vi "AIT 1553 - Parse BC Channels.vi"(6 "Bus Config Info":T10, 7 "FIFO Idx Qs":T12, 8 "error in (no error)":errorcluster, 9 "Bus Page Ref":T1 format="%.0x", 10 "Section GUID":string, 11 "Device Reference in":T1 format="%.0x") -> (0 "error out":errorcluster, 1 "Section BaseRate":u32, 2 "HW Channel - BC Section":T2 {"Message Settings"."Driver Data"."First Word" min=8 max=31; "Message Settings"."Driver Data"."Num Bits" min=1 max=32; "Message Settings"."Driver Data"."Start Bit" min=8 max=31; "Message Settings"."Block Data Refs"."Data Reference" format="%.0x"}, 3 "Device Reference out":T1 format="%.0x", 5 "Bus Controller Page Acyclic Frame Refs out":T1[](array[typedef]) format="%.0x")   [LabVIEW 2013, in "AIT 1553 Custom Device.lvlib"]
uses:
  AIT 1553 Custom Device.lvlib
  <vilib>/NI Veristand/Custom Device API/Custom Device Item Ref.ctl
  RT Controls/FIFO Idx Qs.ctl
  RT Controls/AIT 1553 - Board Config Info.ctl
  RT Controls/AIT 1553 - Hardware Type.ctl
  RT Controls/AIT 1553 - RT HW Channel.ctl
  RT Controls/AIT 1553 - Bus Section.ctl
  RT Controls/AIT 1553 - RT Message Settings.ctl
  <vilib>/NI Veristand/Custom Device API/Block Data Reference.ctl
  <vilib>/NI Veristand/Custom Device API/Data Reference.ctl
  RT Controls/AIT 1553 - Driver Data.ctl
  Controls and Global/Start Bit.ctl
  Controls and Global/Number of Bits.ctl
  <vilib>/NI Veristand/Custom Device Tools/Custom Device Utility Library/RT Debug String Color Spec.ctl
  <vilib>/NI Veristand/Custom Device Tools/Custom Device Utility Library/NI VeriStand - Search for Item by GUID.vi
  Controls and Global/Global.vi
  <vilib>/NI Veristand/Custom Device Tools/Custom Device Utility Library/Custom Device Utility Library.lvlib
  <vilib>/NI Veristand/Custom Device API/Custom Device API.lvlib
  <instrlib>/AIT 1553/AIT 1553.lvlib
  <userlib>/MIL-STD-1553/Owl1553.lvlib
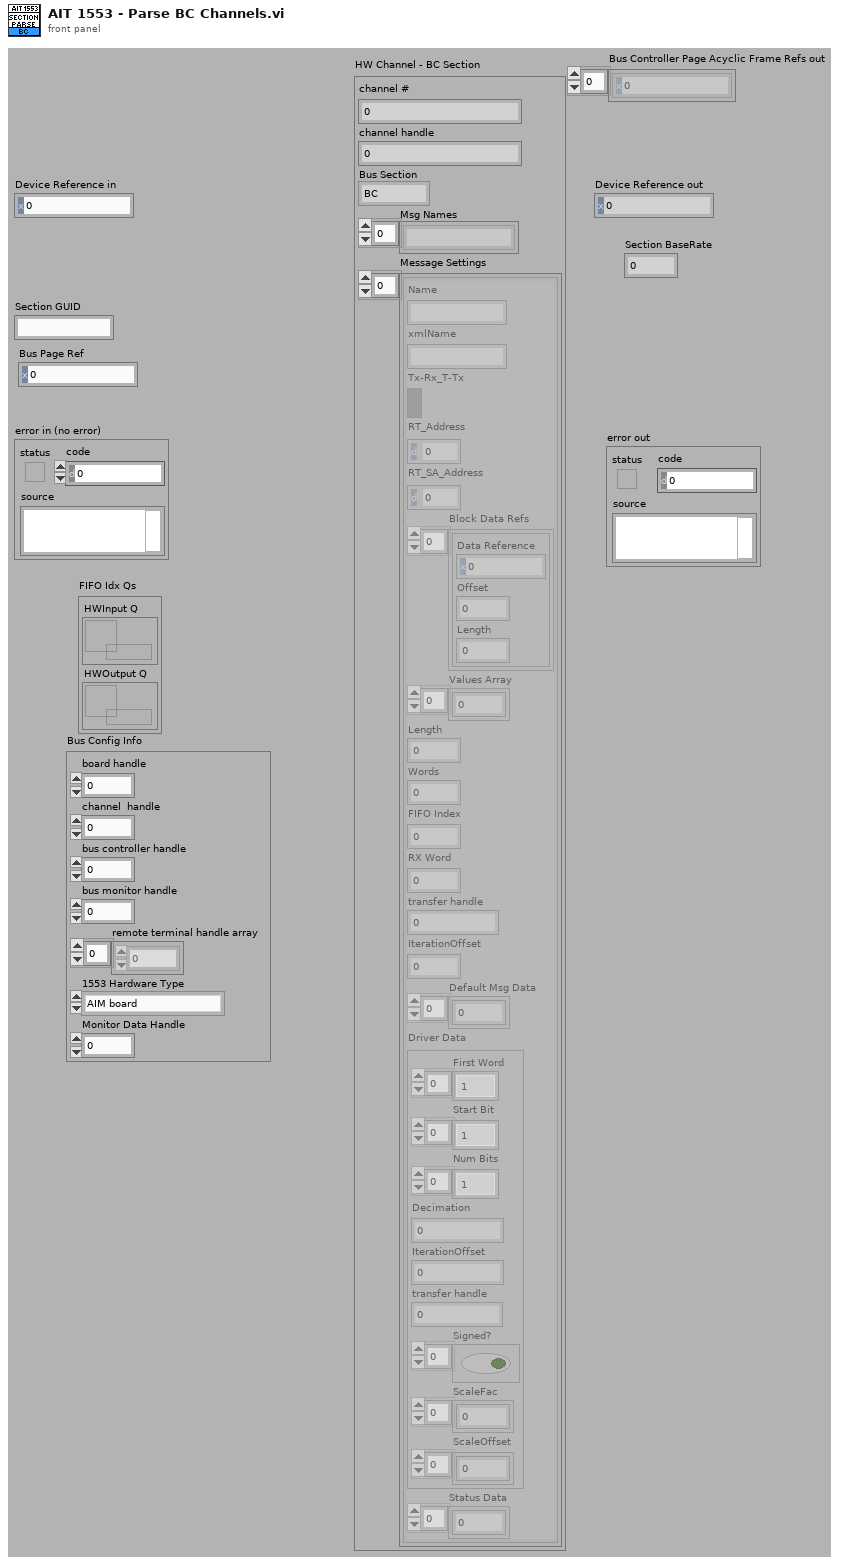
[diagram p1: front panel]
types:
  T1 = typedef "Custom Device API.lvlib/Custom Device Item Ref.ctl" = u64
  T2 = typedef "AIT 1553 Custom Device.lvlib/AIT 1553 - RT HW Channel.ctl" = cluster{"channel #":u16, "channel handle":u32, "Bus Section":T3, "Msg Names":string[], "Message Settings":T4[]}
  T3 = typedef "AIT 1553 Custom Device.lvlib/AIT 1553 - Bus Section.ctl" = enum16{"BC", "BM", "RT"}
  T4 = typedef "AIT 1553 Custom Device.lvlib/AIT 1553 - RT Message Settings.ctl" = cluster{"Name":string, "xmlName":string, "Tx-Rx_T-Tx":bool, "RT_Address":u8, "RT_SA_Address":u8, "Block Data Refs":T5[], "Values Array":dbl[], "Length":i32, "Words":i32, "FIFO Index":i32, "RX Word":u32, "transfer handle":u32, "IterationOffset":i32, "Default Msg Data":u16[], "Driver Data":T7, "Status Data":u32[]}
  T5 = typedef "Custom Device API.lvlib/Block Data Reference.ctl" = cluster{"Data Reference":T6, "Offset":i32, "Length":i32}
  T6 = typedef "Custom Device API.lvlib/Data Reference.ctl" = i32
  T7 = typedef "AIT 1553 Custom Device.lvlib/AIT 1553 - Driver Data.ctl" = cluster{"First Word":T8[], "Start Bit":T8[], "Num Bits":T9[], "Decimation":i32, "IterationOffset":i32, "transfer handle":u32, "Signed?":bool[], "ScaleFac":dbl[], "ScaleOffset":dbl[]}
  T8 = typedef "AIT 1553 Custom Device.lvlib/Start Bit.ctl" = i32
  T9 = typedef "AIT 1553 Custom Device.lvlib/Number of Bits.ctl" = i32
  T10 = typedef "AIT 1553 Custom Device.lvlib/AIT 1553 - Board Config Info.ctl" = cluster{"board handle":u32, "channel  handle":u32, "bus controller handle":u32, "bus monitor handle":u32, "remote terminal handle array":u32[], "1553 Hardware Type":T11, "Monitor Data Handle":u32}
  T11 = typedef "AIT 1553 Custom Device.lvlib/AIT 1553 - Hardware Type.ctl" = enum16{"AIM board", "AIT Board"}
  T12 = typedef "AIT 1553 Custom Device.lvlib/FIFO Idx Qs.ctl" = cluster{"HWInput Q":refnum<queue>, "HWOutput Q":refnum<queue>}
  T13 = typedef "Custom Device Utility Library.lvlib/RT Debug String Color Spec.ctl" = u16
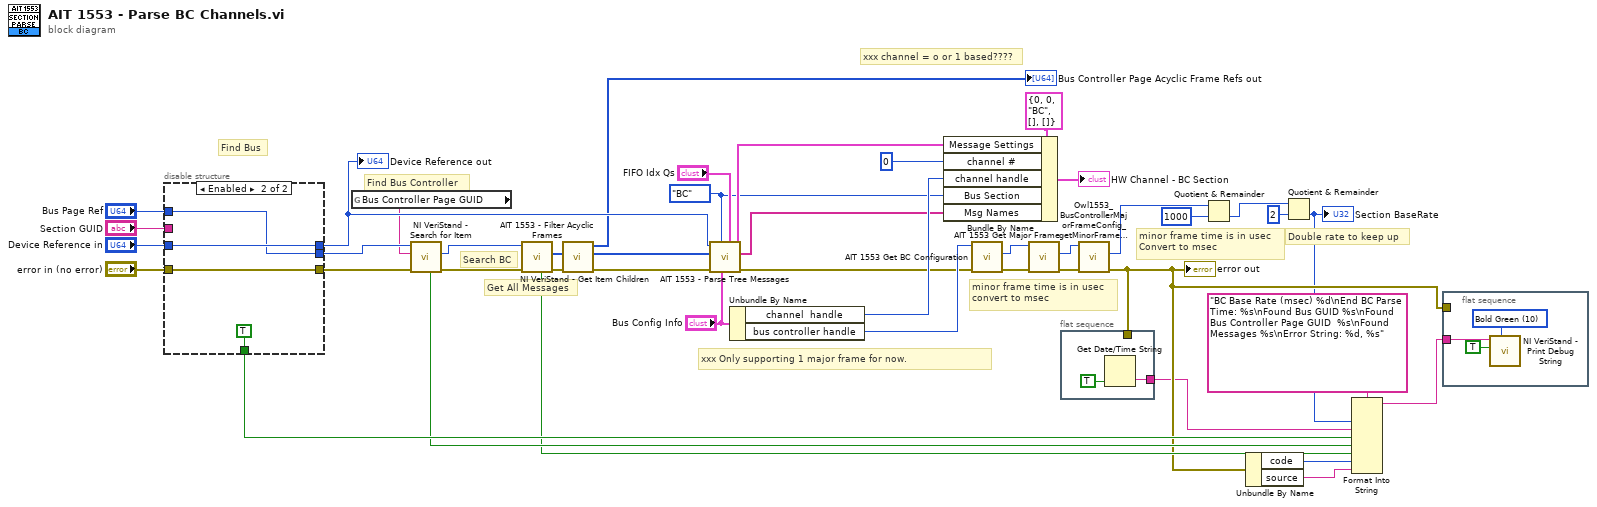
[diagram p0: block diagram]
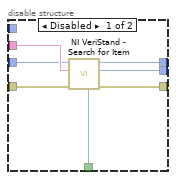
[diagram p2: hidden frame]
diagram:
  w18 = AIT_1553_-_Bus_Section."BC" ("Bus Section")
  # "Double rate to keep up"
  # "xxx channel = o or 1 based????"
  # "minor frame time is in usec\nconvert to msec"
  # "minor frame time is in usec\nConvert to msec"
  # "Find Bus Controller"
  # "Find Bus"
  # "xxx Only supporting 1 major frame for now."
  # "Get All Messages"
  # "Search BC"
  n1 = disable-structure shown="Enabled" {
    disable-tunnel: "Section GUID" -> [w51 _]
    disable-tunnel: "error in (no error)" -> [w50 w54]
    disable-tunnel: [w49 w52] -> w38
    disable-tunnel: [w48 w55] -> w37
    disable-tunnel: [w47 w54] -> w36
    disable-tunnel: [w46 TRUE ("Found")] -> w31
    disable-tunnel: "Device Reference in" -> [w45 w55]
    disable-tunnel: "Bus Page Ref" -> [_ w52]
    frame Disabled {
      n2 = call-poly <vilib>:"NI VeriStand - Search for Item.vi"("error in"=w50, "Item GUID"=w51, "Section Ref in"=w45) -> ("error out"=w47:errorcluster, "Item Ref"=w49:T1, "Section Ref out"=w48:T1, "Found"=w46:bool)  [unwired: 5 in]
    }
    frame Enabled {
    }
  }
  "Device Reference out" <- w37
  n3 = global read "Global.vi" "Bus Controller Page GUID"() -> (w33:string)
  n4 = call-poly <vilib>:"NI VeriStand - Search for Item.vi"("error in"=w36, "Item GUID"=w33, "Section Ref in"=w38) -> ("error out"=w35:errorcluster, "Item Ref"=w34:T1, "Found"=w30:bool)  [unwired: 5 in, 1 out]
  n5 = call <vilib>:"NI VeriStand - Get Item Children.vi"("error in (no error)"=w35, "Item Ref in"=w34) -> ("error out"=w12:errorcluster, "Child Refs"=w10:T1[], "Found"=w27:bool)  [unwired: 6 in, 1 out]
  n6 = call "AIT 1553 - Filter Acyclic Frames.vi"("error in (no error)"=w12, "Bus Controller Page Item Refs in"=w10) -> ("error out"=w11:errorcluster, "Bus Controller Page Message Section Refs out"=w9:T1[], "Bus Controller Page Acyclic Frame Refs out"=→"Bus Controller Page Acyclic Frame Refs out":T1[])  [unwired: 7 in]
  n7 = call "AIT 1553 - Parse Tree Messages.vi"("FIFO Idx Qs"="FIFO Idx Qs", "Bus Config Info"="Bus Config Info", "Bus Section"=w18, "error out"=w11, "Message Refs"=w9, "Custom Device Ref"=w37) -> ("error out"=w4:errorcluster, "Msg Names"=w8:string[], "Message Settings"=w21:T4[])  [unwired: 3 in]
  n8 = Unbundle By Name("Bus Config Info") -> ("channel  handle"=w39:u32, "bus controller handle"=w5:u32)
  n9 = Bundle By Name(cluster=T2 {"channel #"=0, "channel handle"=0, "Bus Section"=enum."BC", "Msg Names"=[], "Message Settings"=[]} ("HW Channel"), "Message Settings"=w21, "channel #"=u16 0, "channel handle"=w39, "Bus Section"=w18, "Msg Names"=w8) -> (→"HW Channel - BC Section":T2)
  n10 = call <instrlib>:"AIT 1553 Get BC Configuration.vi"("error in"=w4, "bus controller handle in"=w5) -> ("error out"=w26:errorcluster, "BC config handle out"=w24:u32)  [unwired: 7 in, 1 out]
  n11 = call <instrlib>:"AIT 1553 Get Major Frame.vi"("error in"=w26, "bus controller config handle in"=w24) -> ("error out"=w25:errorcluster, "major frame config handle out"=w23:u32)  [unwired: 7 in, 1 out]
  n12 = flat-sequence {
    tunnel: [w57] -> w13
    tunnel: w17 -> [_]
    frame #0 {
      n13 = Get Date/Time String(want seconds? (F)=TRUE) -> (time string=w57:string)  [unwired: 2 in, 1 out]
    }
  }
  n14 = call <userlib>:"Owl1553_BusControllerMajorFrameConfig_getMinorFrameTime.vi"("error in (no error)"=w25, "config handle"=w23) -> ("error out"=w17:errorcluster, "minor frame time"=w16:u32)  [unwired: 7 in, 1 out]
  "error out" <- w17
  n15 = Quotient & Remainder(x=w16, y=u32 1000) -> (floor(x/y)=w14:u32)  [unwired: 1 out]
  n16 = Unbundle By Name(w17) -> ("code"=w28:i32, "source"=w1:string)
  n17 = Quotient & Remainder(x=w14, y=u32 2) -> (floor(x/y)=w2:u32)  [unwired: 1 out]
  "Section BaseRate" <- w2
  n18 = Format Into String(format string="BC Base Rate (msec) %d\nEnd BC Parse Time: %s\nFound Bus GUID %s\nFound Bus Controller Page GUID  %s\nFound Messages %s\nError String: %d, %s", w2, w13, w31, w30, w27, w28, w1) -> (resulting string=w32:string)  [unwired: 2 in, 1 out]
  n19 = flat-sequence {
    tunnel: w32 -> [w59]
    tunnel: w17 -> [_]
    frame #0 {
      w60 = T13 10 items=["Plain White"=7, "Bold White"=15, "Bold Blue"=9, "Bold Green"=10, "Bold Red"=12] ("Attribute")
      n20 = call <vilib>:"NI VeriStand - Print Debug String.vi"("Attribute"=w60, "Add to log file? (T)"=TRUE, "Message"=w59) -> ()  [unwired: 8 in, 1 out]
    }
  }
